vi "Initial Values-format and values-Ref select window.vi"() -> (13 "Values.Boolean":bool[](array[boolean]), 14 "Keys setup.DBL":T2=[{"key"="Control FPGA.Clock Freq (MHz)", "Save?"=TRUE, "Default"=240.0}, {"key"="DAQ FPGA.Clock Freq (MHz)", "Save?"=TRUE, "Default"=240.0}], 15 "Values.DBL":dbl[](array[numeric]), 16 "Keys setup.String":T3=[{"key"="Control FPGA.MAC address", "Save?"=TRUE, "Default"="AABBCCDDEEFF"}, {"key"="DAQ FPGA.Target", "Save?"=TRUE, "Default"="RIO0"}, {"key"="XY Stage.COM port", "Save?"=TRUE, "Default"="COM7"}, {"key"="DAQmx Chan.Pockels Control", "Save?"=TRUE, "Default"=""}, {"key"="DAQmx Chan.Hard Shutter", "Save?"=TRUE, "Default"=""}, {"key"="DAQmx Chan.PMT 1", "Save?"=TRUE, "Default"=""}, {"key"="DAQmx Chan.PMT 2", "Save?"=TRUE, "Default"=""}, {"key"="DAQmx Chan.Encoder Trigger", "Save?"=TRUE, "Default"=""}, {"key"="DAQmx Chan.Optional Trigger 1", "Save?"=TRUE, "Default"=""}, {"key"="DAQmx Chan.Optional Trigger 2", "Save?"=TRUE, "Default"=""}, {"key"="DAQmx Chan.Optional Trigger 3", "Save?"=TRUE, "Default"=""}], 17 "Values.Strings":string[](array[string]), 18 "Keys setup.Boolean":T1, 19 "error out":errorcluster)   [LabVIEW 2020]
uses:
  Typedefs/Ini file interface (String).ctl
  Typedefs/Ini file interface (DBL).ctl
  Typedefs/Ini file interface (Boolean).ctl
  User Interface/Globals/gl_Windows Ctrl refs.vi
panel:
  # "NOTES:\n1. \"Control FPGA.Ethernet port\" is detected automatically. It is not saved/loaded from file.\n2. \"Control FPGA.Ethernet Opened\" is detected automatically. It is not saved/loaded from file."
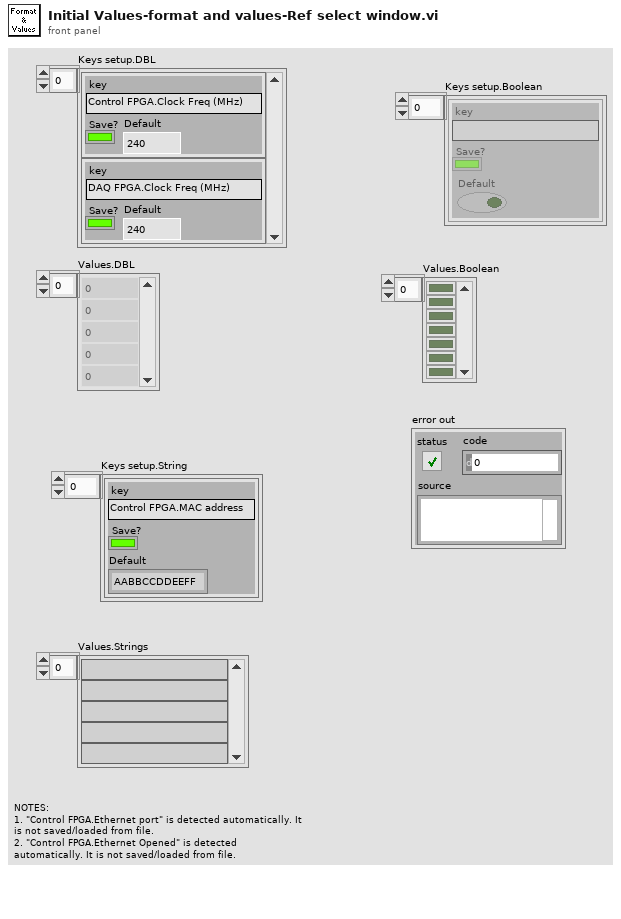
[diagram p1: front panel]
types:
  T1 = typedef "Ini file interface (Boolean).ctl" = cluster{"key":string, "Save?":bool, "Default":bool}[]
  T2 = typedef "Ini file interface (DBL).ctl" = cluster{"key":string, "Save?":bool, "Default":dbl}[]
  T3 = typedef "Ini file interface (String).ctl" = cluster{"key":string, "Save?":bool, "Default":string}[]
  T4 = typedef "Ref select window ctrl refs.ctl" = cluster{"Channel Selector":refnum<vi>, "Boundary":refnum<vi>, "Image intensity":refnum<vi>}
  T5 = typedef "Channel Selector.ctl" = enum16{"Red Channel", "Green Channel", "Blended"}
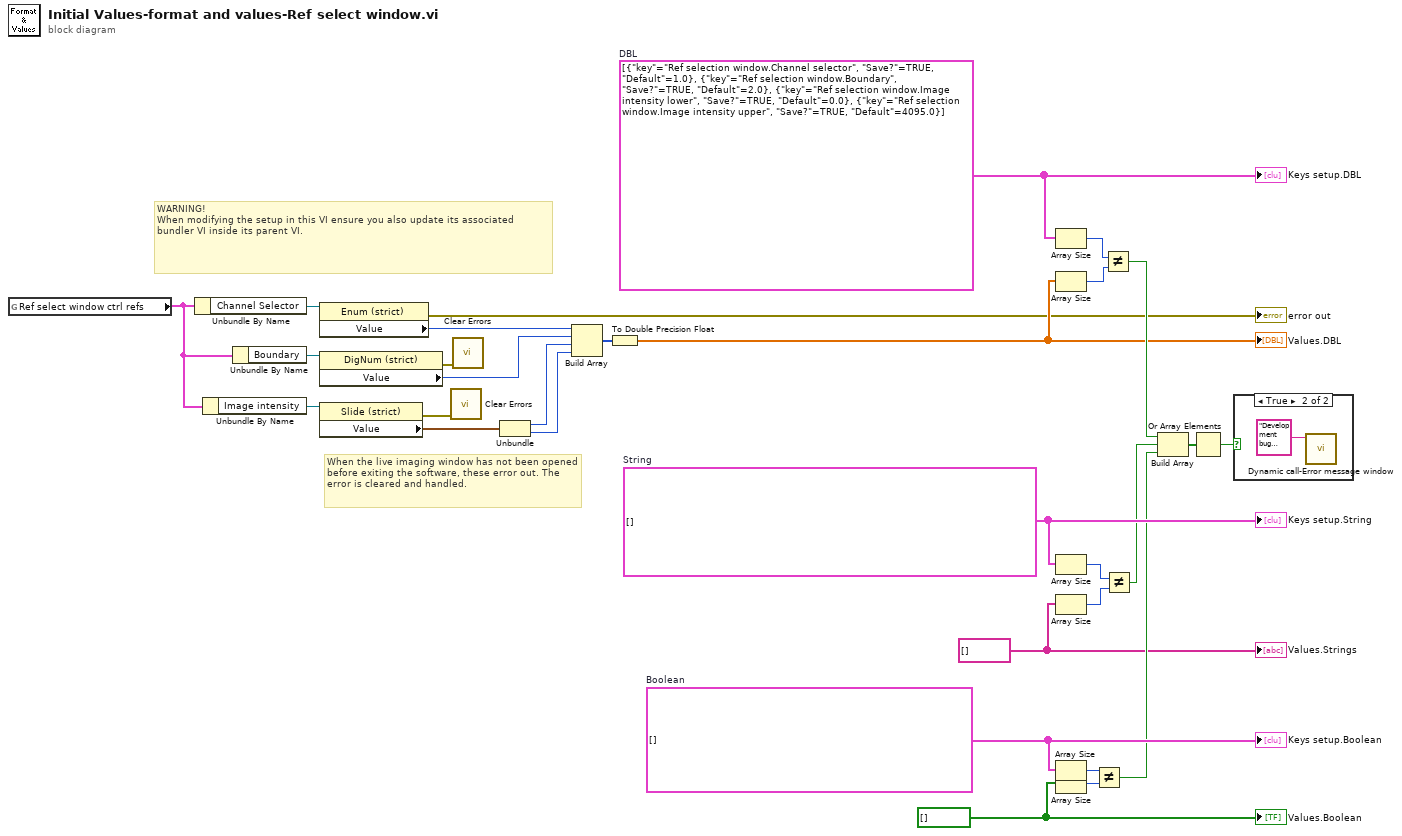
[diagram p0: block diagram]
diagram:
  w13 = string[] [] ("appended array")
  w14 = bool[] [] ("appended array")
  w27 = T1 []  # Boolean
  w30 = T3 []  # String
  w29 = T2 [{"key"="Ref selection window.Channel selector", "Save?"=TRUE, "Default"=1.0}, {"key"="Ref selection window.Boundary", "Save?"=TRUE, "Default"=2.0}, {"key"="Ref selection window.Image intensity lower", "Save?"=TRUE, "Default"=0.0}, {"key"="Ref selection window.Image intensity upper", "Save?"=TRUE, "Default"=4095.0}]  # DBL
  # "When the live imaging window has not been opened before exiting the software, these error out. The error is cleared and handled."
  # "WARNING!\nWhen modifying the setup in this VI ensure you also update its associated bundler VI inside its parent VI."
  n1 = global read "gl_Windows Ctrl refs.vi" "Ref select window ctrl refs"() -> (w1:T4)
  n2 = Unbundle By Name(w1) -> ("Channel Selector"=w15:refnum<vi>)
  n3 = Unbundle By Name(w1) -> ("Image intensity"=w8:refnum<vi>)
  n4 = Unbundle By Name(w1) -> ("Boundary"=w11:refnum<vi>)
  n5 = property class="Enum (strict)"(reference=w15) -> (error out=→"error out":errorcluster, "Value"=w12:T5)  [unwired: 1 in, 1 out]
  n6 = property class="DigNum (strict)"(reference=w11) -> (error out=w6:errorcluster, "Value"=w10:i16)  [unwired: 1 in, 1 out]
  n7 = property class="Slide (strict)"(reference=w8) -> (error out=w5:errorcluster, "Value"=w7:cluster{i16, i16})  [unwired: 1 in, 1 out]
  n8 = call <vilib>:"Clear Errors.vi"("error in (no error)"=w5) -> ()  [unwired: 5 in, 2 out]
  n9 = call <vilib>:"Clear Errors.vi"("error in (no error)"=w6) -> ()  [unwired: 5 in, 2 out]
  n10 = Unbundle(w7) -> (w3:i16, w2:i16)
  n11 = Build Array(w12, w10, w3, w2) -> (w28:u16[])
  n12 = To Double Precision Float(number=w28) -> (double precision float=w9:dbl[])
  "Values.DBL" <- w9
  n13 = Array Size(array=w29) -> (size(s)=w24:i32)
  n14 = Array Size(array=w9) -> (size(s)=w23:i32)
  n15 = Array Size(array=w30) -> (size(s)=w26:i32)
  n16 = Array Size(array=w13) -> (size(s)=w25:i32)
  n17 = Array Size(array=w27) -> (size(s)=w22:i32)
  n18 = Array Size(array=w14) -> (size(s)=w21:i32)
  n19 = Not Equal?(x=w22, y=w21) -> (x != y?=w19:bool)
  n20 = Not Equal?(x=w24, y=w23) -> (x != y?=w17:bool)
  n21 = Not Equal?(x=w26, y=w25) -> (x != y?=w16:bool)
  n22 = Build Array(w17, w16, w19) -> (w20:bool[])
  n23 = Or Array Elements(Boolean array=w20) -> (logical OR=w18:bool)
  n24 = case shown="True" w18 {
    frame False {
    }
    frame True {
      n25 = call "Dynamic call-Error message window.vi"("Error Message"="Development bug detected in the \"Initial Values-format and values-Ref select window.vi\".\nPlease correct the set up in this VI.") -> ()  [unwired: 10 in, 1 out]
    }
  }
  "Keys setup.String" <- w30
  "Keys setup.DBL" <- w29
  "Values.Strings" <- w13
  "Keys setup.Boolean" <- w27
  "Values.Boolean" <- w14
